vi "Wait for Acquisition Complete.vi"(8 "error in (no error)":errorcluster, 10 "Maximum Time (10000 ms)":u32=10000, 11 "VISA resource name":refnum<visa-resource-name>) -> (0 "error out":errorcluster, 3 "VISA resource name out":refnum<visa-resource-name>)   [LabVIEW 2015, in "Template - Counter.lvlib"]
doc: "Waits for the current acquisition to finish. This VI should be called after <b>Initiate</b> VI and before <b>Fetch</b> VI.\n\n<B>Note:</B> \n\nUse this VI only with other low-level VIs. The high-level VIs automatically incorporate this functionality. This VI does not check the instrument status."
uses:
  <instrlib>/_Template - Counter/Template - Counter.lvlib
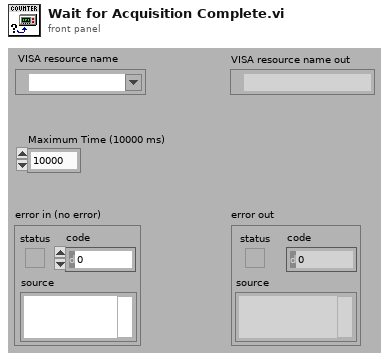
[diagram p1: front panel]
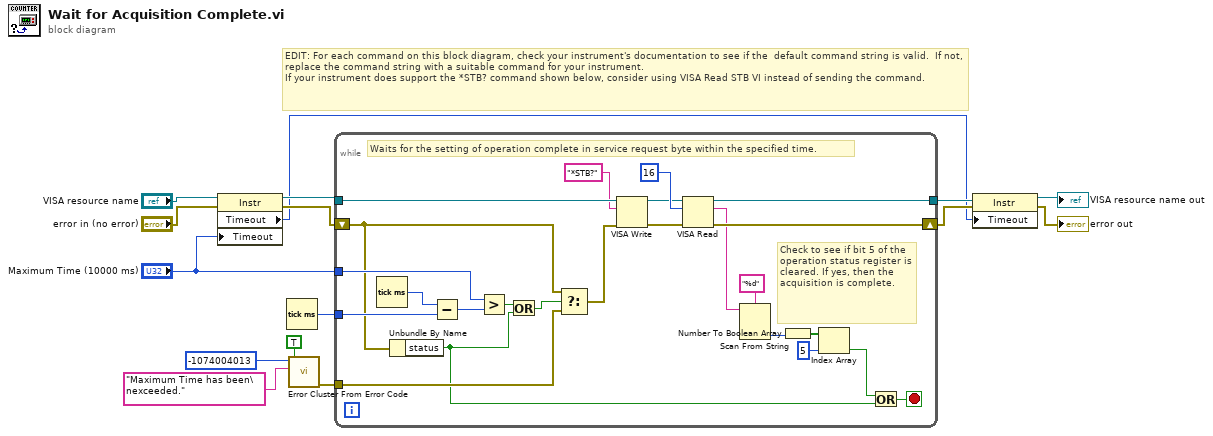
[diagram p0: block diagram]
diagram:
  # "EDIT: For each command on this block diagram, check your instrument's documentation to see if the  default command string is valid.  If not, replace the command string with a suitable command for your instrument. \nIf your instrument does support the *STB? command shown below, consider using VISA Read STB VI instead of sending the command."
  n1 = property class="Instr"(reference="VISA resource name", error in="error in (no error)", "Timeout"="Maximum Time (10000 ms)") -> (reference out=w5:refnum<visa-resource-name>, error out=w3:errorcluster, "Timeout"=w1:u32)
  n2 = Tick Count (ms)() -> (millisecond timer value=w12:u32)
  n3 = call <vilib>:"Error Cluster From Error Code.vi"("show call chain? (False)"=TRUE, "error message (\"\")"="Maximum Time has been\nexceeded." ("error message (\"\")"), "error code (0)"=-1074004013) -> ("error out"=w11:errorcluster)  [unwired: 6 in]
  n4 = while {
    tunnel: [w38] -> w9
    tunnel: w5 -> [w37]
    tunnel: "Maximum Time (10000 ms)" -> [w33]
    tunnel: w12 -> [w34]
    tunnel: w11 -> [w30]
    shift-right: [w39] -> w10
    shift-left: w3 -> [w31]
    stop <- w27 stop-if-true
    # "Waits for the setting of operation complete in service request byte within the specified time."
    # "Check to see if bit 5 of the operation status register is cleared. If yes, then the acquisition is complete."
    n5 = Tick Count (ms)() -> (millisecond timer value=w36:u32)
    n6 = Unbundle By Name(w31) -> ("status"=w17:bool)
    n7 = Subtract(x=w36, y=w34) -> (x-y=w35:u32)
    n8 = Greater?(x=w33, y=w35) -> (0:w16:bool)
    n9 = Or(x=w16, y=w17) -> (x .or. y?=w32:bool)
    n10 = Select(t=w31, s=w32, f=w30) -> (s? t:f=w29:errorcluster)
    n11 = VISA Write(VISA resource name=w37, write buffer="*STB?", error in (no error)=w29) -> (VISA resource name out=w21:refnum<visa-resource-name>, error out=w22:errorcluster)  [unwired: 1 out]
    n12 = VISA Read(VISA resource name=w21, byte count=u32 16, error in (no error)=w22) -> (VISA resource name out=w38:refnum<visa-resource-name>, read buffer=w26:string, error out=w39:errorcluster)  [unwired: 1 out]
    n13 = Scan From String(format string="%d", input string=w26) -> (output 1=w18:i32)  [unwired: 3 in, 3 out]
    n14 = Number To Boolean Array(number=w18) -> (Boolean array=w20:bool[])
    n15 = Index Array(array=w20, index=5) -> (element=w28:bool)
    n16 = Or(x=w28, y=w17) -> (x .or. y?=w27:bool)
  }
  n17 = property class="Instr"(reference=w9, error in=w10, "Timeout"=w1) -> (reference out=→"VISA resource name out":refnum<visa-resource-name>, error out=→"error out":errorcluster)
